vi "Read Future.vi"(6 "Top Future":refnum<class "Future.lvclass">, 7 "Top Level?":bool, 8 "error in (no error)":errorcluster, 9 "timeout in ms (-1)":i32=-1, 11 "Future in":refnum<class "Future.lvclass">) -> (0 "error out":errorcluster, 1 "timed out?":bool, 2 "Value":variant, 3 "Future out":refnum<class "Future.lvclass">)   [LabVIEW 2017, in "Promise Future.lvlib" / "Future.lvclass"]
uses:
  Future.lvclass
  Future.lvclass/Future.ctl
  Rejected Future/Rejected Future.lvclass
  E:/Promise/Promise Future/Future/Future.lvclass
  Rejected Future/Rejected Future.lvclass/Rejected Future.ctl
  Rejected Future/Read Reason.vi
  <vilib>/Utility/error.llb/Error Cluster From Error Code.vi
  <vilib>/ErrorRing/Error Ring.xnode
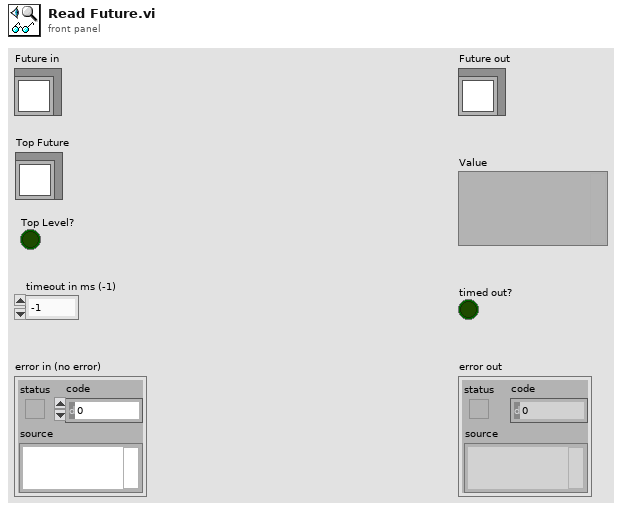
[diagram p1: front panel]
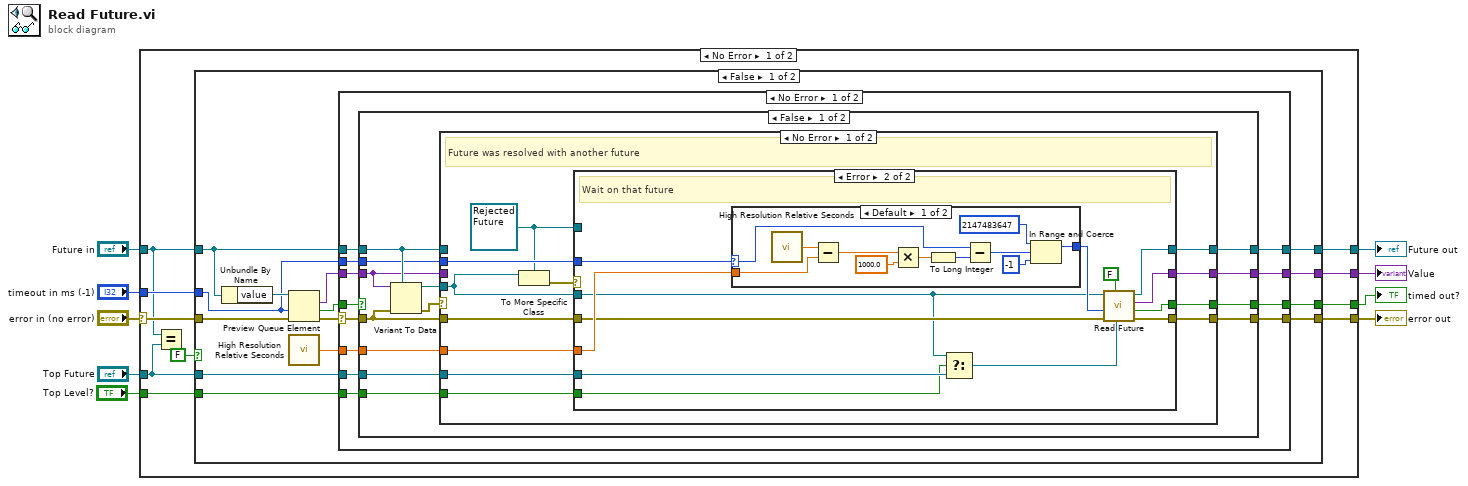
[diagram p0: block diagram]
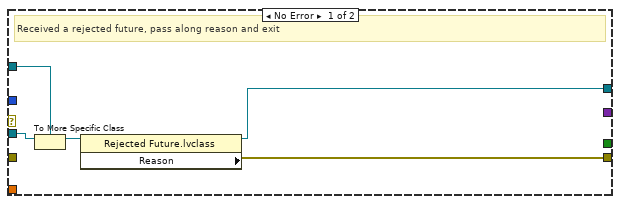
[diagram p2: hidden frame]
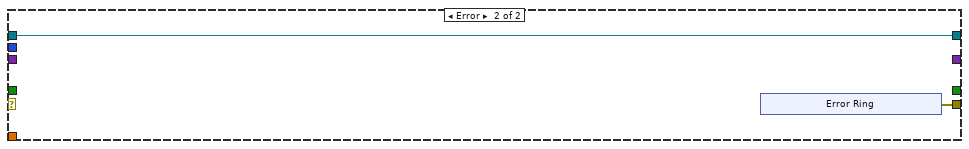
[diagram p6: hidden frame]
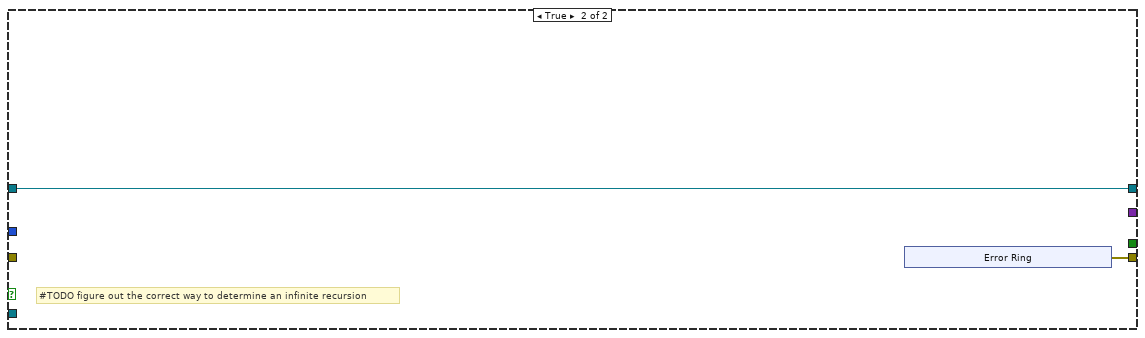
[diagram p7: hidden frame]
diagram:
  n1 = case shown="No Error" "error in (no error)" {
    selector: "error in (no error)" -> [w19 w123]
    tunnel: [w17 w123] -> w4
    tunnel: [w15 w122] -> w3
    tunnel: "Future in" -> [w13 w122]
    tunnel: [w16 _] -> w5
    tunnel: [w18 _] -> w6
    tunnel: "timeout in ms (-1)" -> [w14 _]
    tunnel: "Top Future" -> [w12 _]
    tunnel: "Top Level?" -> [w11 _]
    frame No Error {
      n2 = Equal?(x=w13, y=w12) -> ()  [unwired: 1 out]
      n3 = case shown="False" FALSE {
        tunnel: w19 -> [w32 _]
        tunnel: [w28 _] -> w18
        tunnel: [w27 w115] -> w17
        tunnel: [w26 _] -> w16
        tunnel: w13 -> [w25 w116]
        tunnel: [w24 w116] -> w15
        tunnel: w14 -> [w23 _]
        tunnel: w12 -> [w21 _]
        tunnel: w11 -> [w20 _]
        frame False {
          n4 = Unbundle By Name(w25) -> ("value"=w33:refnum<queue>)
          n5 = Preview Queue Element(queue=w33, timeout in ms (-1)=w23, error in (no error)=w32) -> (element=w30:variant, timed out?=w31:bool, error out=w29:errorcluster)  [unwired: 1 out]
          n6 = call <vilib>:"High Resolution Relative Seconds.vi"() -> ("relative seconds"=w22:dbl)
          n7 = case shown="No Error" w29 {
            selector: w29 -> [w43 _]
            tunnel: w31 -> [w45 _]
            tunnel: w30 -> [w44 _]
            tunnel: [w42 _] -> w28
            tunnel: [w41 w109] -> w27
            tunnel: [w40 _] -> w26
            tunnel: w25 -> [w39 w108]
            tunnel: [w38 w108] -> w24
            tunnel: w23 -> [w37 _]
            tunnel: w22 -> [w36 _]
            tunnel: w21 -> [w35 _]
            tunnel: w20 -> [w34 _]
            frame No Error {
              n8 = case shown="False" w45 {
                selector: w45 -> [_ w105]
                tunnel: w44 -> [w50 w107]
                tunnel: w43 -> [w57 w106]
                tunnel: [w58 w107] -> w42
                tunnel: [w56 w106] -> w41
                tunnel: [w54 w105] -> w40
                tunnel: w39 -> [w53 w104]
                tunnel: [w52 w104] -> w38
                tunnel: w36 -> [w49 _]
                tunnel: w37 -> [w48 _]
                tunnel: w35 -> [w47 _]
                tunnel: w34 -> [w46 _]
                frame False {
                  n9 = Variant To Data(error in=w57, type=w53, Variant=w50) -> (data=w51:refnum<class "Future.lvclass">, error out=w55:errorcluster)
                  n10 = case shown="No Error" w55 {
                    tunnel: [w70 w101] -> w58
                    tunnel: w57 -> [w63 w103]
                    tunnel: [w68 w103] -> w56
                    tunnel: [w69 _] -> w54
                    tunnel: w53 -> [_ w102]
                    tunnel: [w61 w102] -> w52
                    tunnel: w51 -> [w64 _]
                    tunnel: w50 -> [_ w101]
                    tunnel: w49 -> [w66 _]
                    tunnel: w48 -> [w67 _]
                    tunnel: w47 -> [w60 _]
                    tunnel: w46 -> [w59 _]
                    frame No Error {
                      w62 = refnum<class "Rejected Future.lvclass"> refnum ("Promise Future.lvlib:Rejected Future.lvclass")
                      # "Future was resolved with another future"
                      n11 = To More Specific Class(target class=w62, reference=w64) -> (error out=w65:errorcluster)  [unwired: 1 in, 1 out]
                      n12 = case shown="Error" w65 {
                        tunnel: [_ w84] -> w70
                        tunnel: [_ w85] -> w69
                        tunnel: [w71 w86] -> w68
                        tunnel: w67 -> [_ w88]
                        tunnel: w66 -> [_ w87]
                        tunnel: w64 -> [w75 w80]
                        tunnel: w62 -> [w74 _]
                        tunnel: w63 -> [_ w82]
                        tunnel: [w72 w81] -> w61
                        tunnel: w60 -> [_ w79]
                        tunnel: w59 -> [_ w76]
                        frame No Error {
                          # "Received a rejected future, pass along reason and exit"
                          n13 = To More Specific Class(target class=w74, reference=w75) -> (specific class reference=w73:refnum<class "Rejected Future.lvclass">)  [unwired: 1 in, 1 out]
                          n14 = property class="Rejected Future.lvclass"(reference=w73) -> (reference out=w72:refnum<class "Rejected Future.lvclass">, "Reason"=w71:errorcluster)  [unwired: 1 in, 1 out]
                        }
                        frame Error {
                          # "Wait on that future"
                          n15 = case shown="Default" w88 {
                            selector: w88 -> [w99 w100]
                            tunnel: w87 -> [w97 _]
                            tunnel: [w91 w100] -> w83
                            frame Default {
                              n16 = call <vilib>:"High Resolution Relative Seconds.vi"() -> ("relative seconds"=w98:dbl)
                              n17 = Subtract(x=w98, y=w97) -> (x-y=w96:dbl)
                              n18 = Multiply(x=w96, y=1000.0 ("x")) -> (x*y=w94:dbl)
                              n19 = To Long Integer(number=w94) -> (32bit integer=w93:i32)
                              n20 = Subtract(x=w99, y=w93) -> (x-y=w92:i32)
                              n21 = In Range and Coerce(upper limit=2147483647, x=w92, lower limit=-1) -> (coerced(x)=w91:i32)  [unwired: 1 out]
                            }
                            frame -1, 0 {
                            }
                          }
                          n22 = Select(t=w80, s=w76, f=w79) -> (s? t:f=w78:refnum<class "Future.lvclass">)
                          n23 = call "Read Future.vi"("Top Future"=w78, "Top Level?"=FALSE, "error in (no error)"=w82, "timeout in ms (-1)"=w83, "Future in"=w80) -> ("error out"=w86:errorcluster, "timed out?"=w85:bool, "Value"=w84:variant, "Future out"=w81:refnum<class "Future.lvclass">)  [unwired: 3 in]
                        }
                      }
                    }
                    frame Error {
                      # "Just a normal value, pass it along"
                    }
                  }
                }
                frame True {
                }
              }
            }
            frame Error {
              n24 = xnode "Error Ring"() -> ("error out"=w109:errorcluster)
            }
          }
        }
        frame True {
          # "#TODO figure out the correct way to determine an infinite recursion"
          n25 = xnode "Error Ring"() -> ("error out"=w115:errorcluster)
        }
      }
    }
    frame Error {
    }
  }
  "error out" <- w4
  "Future out" <- w3
  "Value" <- w6
  "timed out?" <- w5
